vi "_System Locations.vi"() -> (3 "SystemLocations":cluster{"Token":string, "Path":path}[](array[cluster]))   [LabVIEW 2017, in "lvcsm File Support.lvlib"]
uses:
  lvcsm File Support.lvlib
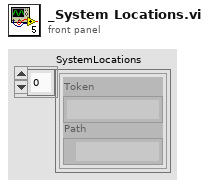
[diagram p1: front panel]
types:
  T1 = cluster{"replace string (\"\")":string, "stripped path":path}[]
  T2 = cluster{"replace string (\"\")":string, "stripped path":path}
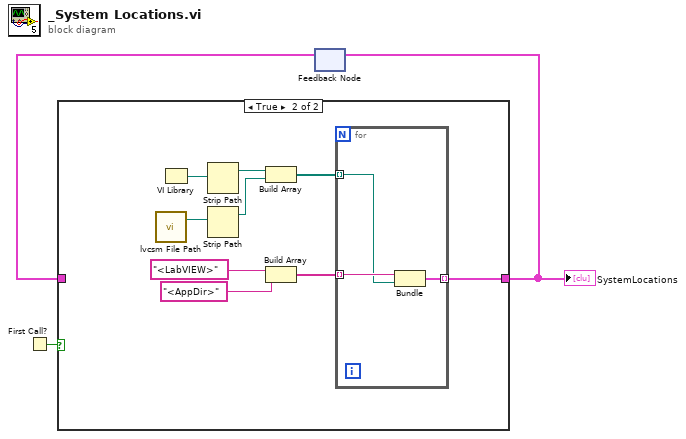
[diagram p0: block diagram]
diagram:
  n1 = First Call?() -> (First Call?: T/F=w1:bool)
  n2 = feedback #1() -> (w2:T1)  [unwired: 1 in]
  n3 = case shown="True" w1 {
    tunnel: [w4 w7] -> w3
    tunnel: w2 -> [w4 _]
    frame False {
    }
    frame True {
      n4 = call "lvcsm File Path.vi"() -> ("Appended Path"=w6:path)  [unwired: 3 in]
      n5 = VI Library() -> (path=w13:path)
      n6 = Strip Path(path=w13) -> (stripped path=w12:path)  [unwired: 1 out]
      n7 = Strip Path(path=w6) -> (stripped path=w5:path)  [unwired: 1 out]
      n8 = Build Array(w12, w5) -> (w8:path[])
      n9 = Build Array("<LabVIEW>" ("replace string (\"\")"), "<AppDir>" ("replace string (\"\")")) -> (w9:string[])
      n10 = for {
        tunnel: w9 -> [w16] mode=indexing
        tunnel: w8 -> [w15] mode=indexing
        tunnel: [w14] -> w7 mode=indexing
        n11 = Bundle("replace string (\"\")"=w16, "stripped path"=w15) -> (w14:T2)  [unwired: 1 in]
      }
    }
  }
  "SystemLocations" <- w3
  n12 = feedback-in #1(w3) -> ()
